vi "Get RUS app refs.vi"(11 "RUS Measurement in":refnum<class "RUS Measurement.lvclass">) -> (0 "error out":errorcluster, 3 "RUS Measurement out":refnum<class "RUS Measurement.lvclass">)   [LabVIEW 2014]
doc: "(<B>Filename</B>: Actor Framework.lvlib:Actor.lvclass:Pre Launch Init.vi)\n\nDefines behavior that occurs after the Launch Actor method is invoked but before the actor's Actor Core method begins running.\n\nThe Pre Launch Init method is guaranteed to finish before the Launch Actor method returns to its caller and before the actor itself receives any messages. Any references that the Pre Launch Init method obtains are guaranteed to have the same lifetime as the actor itself. Any errors that the Pre Launch Init method returns will abort the launch.\n\nBy default, this method does nothing. A descendant class may override it to define behavior."
uses:
  RUS Measurement.lvclass
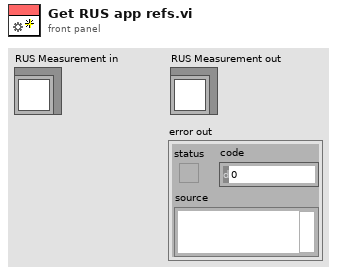
[diagram p1: front panel]
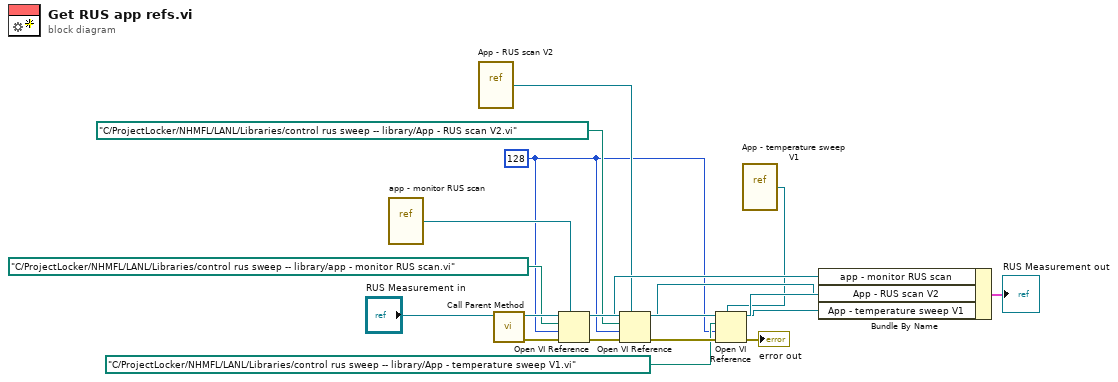
[diagram p0: block diagram]
diagram:
  w3 = 128 ("options")
  n1 = vi-ref "app - monitor RUS scan.vi"() -> (w9:refnum<vi>)
  n2 = vi-ref "App - RUS scan V2.vi"() -> (w8:refnum<vi>)
  n3 = call-parent "Call Parent Method"("Mag Lab Measurement in"="RUS Measurement in") -> ("error out"=w12:errorcluster, "Mag Lab Measurement out"=w17:refnum<class "RUS Measurement.lvclass">)  [unwired: 9 in]
  n4 = Open VI Reference(type specifier VI Refnum (for type only)=w9, vi path=path "C:/ProjectLocker/NHMFL/LANL/Libraries/control rus sweep -- library/app - monitor RUS scan.vi", options=w3, error in (no error)=w12) -> (vi reference=w13:refnum<vi>, error out=w11:errorcluster)  [unwired: 2 in]
  n5 = Open VI Reference(type specifier VI Refnum (for type only)=w8, vi path=path "C:/ProjectLocker/NHMFL/LANL/Libraries/control rus sweep -- library/App - RUS scan V2.vi", options=w3, error in (no error)=w11) -> (vi reference=w7:refnum<vi>, error out=w6:errorcluster)  [unwired: 2 in]
  n6 = vi-ref "App - temperature sweep V1.vi"() -> (w1:refnum<vi>)
  n7 = Open VI Reference(type specifier VI Refnum (for type only)=w1, vi path=path "C:/ProjectLocker/NHMFL/LANL/Libraries/control rus sweep -- library/App - temperature sweep V1.vi", options=w3, error in (no error)=w6) -> (vi reference=w2:refnum<vi>, error out=→"error out":errorcluster)  [unwired: 2 in]
  n8 = Bundle By Name(cluster=w17, "app - monitor RUS scan"=w13, "App - RUS scan V2"=w7, "App - temperature sweep V1"=w2) -> (→"RUS Measurement out":cluster{})
